vi "rectangleBox.vi"(1 "Rectangles 2":T2(array[cluster])) -> (0 "output cluster":T1)   [LabVIEW 2023]
doc: "Used for detecting squares in an image."
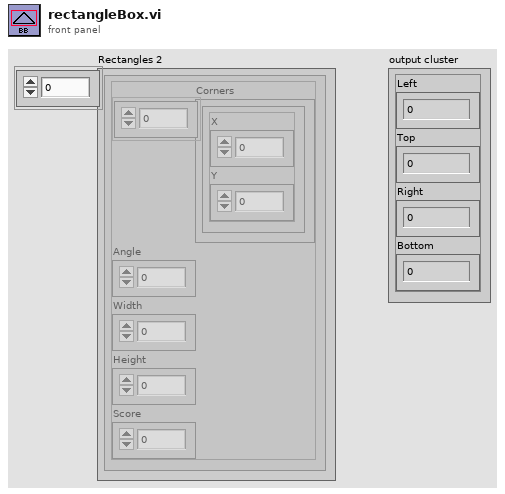
[diagram p1: front panel]
types:
  T1 = cluster{"Left":i32, "Top":i32, "Right":i32, "Bottom":i32}
  T2 = cluster{"Corners":cluster{"X":sgl, "Y":sgl}[], "Angle":dbl, "Width":dbl, "Height":dbl, "Score":dbl}[]
  T3 = cluster{"Corners":cluster{"X":sgl, "Y":sgl}[], "Angle":dbl, "Width":dbl, "Height":dbl, "Score":dbl}
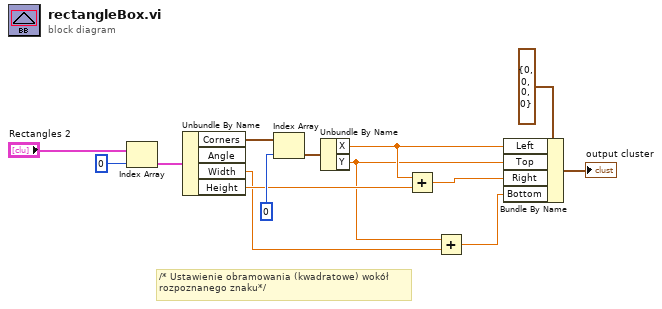
[diagram p0: block diagram]
diagram:
  # "/* Ustawienie obramowania (kwadratowe) wokół rozpoznanego znaku*/"
  n1 = Index Array(array="Rectangles 2", index=0) -> (element=w13:T3)
  n2 = Unbundle By Name(w13) -> ("Corners"=w12:cluster{"X":sgl, "Y":sgl}[], "Width"=w4:dbl, "Height"=w5:dbl)  [unwired: 1 out]
  n3 = Index Array(array=w12, index=0) -> (element=w10:cluster{"X":sgl, "Y":sgl})
  n4 = Unbundle By Name(w10) -> ("X"=w8:sgl, "Y"=w1:sgl)
  n5 = Add(x=w8, y=w5) -> (x+y=w7:dbl)
  n6 = Add(x=w1, y=w4) -> (x+y=w6:dbl)
  n7 = Bundle By Name(cluster=T1 {"Left"=0, "Top"=0, "Right"=0, "Bottom"=0} ("Rectangle"), "Left"=w8, "Top"=w1, "Right"=w7, "Bottom"=w6) -> (→"output cluster":T1)
